vi "9024_8_9230.vi"() -> (2 "Device":T3={"Id"="55379f6619257936b04df56a", "Name"="Tms9024", "DeviceType"="CMS-9024", "HardwareName"="", "IpAddress"="10.2.64.47", "HardwareInfo"=[{"Key"="Controller", "Value"="cRIO 9024"}, {"Key"="Slot 1", "Value"="NI 9232 Tachometer"}, {"Key"="Slot 2", "Value"="NI 9230"}, {"Key"="Slot 3", "Value"="NI 9230"}, {"Key"="Slot 4", "Value"="NI 9230"}, {"Key"="Slot 5", "Value"="NI 9230"}, {"Key"="Slot 6", "Value"="NI 9230"}, {"Key"="Slot 7", "Value"="NI 9230"}, {"Key"="Slot 8", "Value"="NI 9230"}], "ApplicationType"="", "ApplicationVersion"="", "EquipmentIds"=[], "ConfigurationVersion"="2015-04-22T08:26:15.5019992-05:00", "ConfigurationBag"="", "Properties"=[{"Key"="FileMemoryTransferMode", "Value"="true"}, {"Key"="StreamMode", "Value"="InMemOrDisk"}, {"Key"="TdmsMemoryBlockSize", "Value"="8388608"}, {"Key"="TdmsMemoryStreamBlockSize", "Value"="1048576"}, {"Key"="ReconnectInterval", "Value"="30"}, {"Key"="PacketSizeKbytes", "Value"="16"}, {"Key"="InterPacketDelay", "Value"="0"}, {"Key"="FeatureSpeedCutoff", "Value"="120"}, {"Key"="SpeedReference", "Value"=""}, {"Key"="DataBlockLength", "Value"="4"}, {"Key"="DataBlockUnit", "Value"="Seconds"}, {"Key"="AcquisitionLength", "Value"="7"}, {"Key"="PreTriggerLength", "Value"="3"}, {"Key"="AcquisitionUnit", "Value"="Seconds"}], "DataGroups"=[{"Name"="Default", "ChannelIds"=["55379f6619257936b04df56b", "55379f6619257936b04df56e", "55379f6619257936b04df571", "55379f6619257936b04df574", "55379f6619257936b04df579", "55379f6619257936b04df57e"], "GatingTrigger"={"Type"="", "Expression"="", "Conditions"=[]}, "OperatingStates"=[{"Id"="55379f6619257936b04df59b", "Name"="SteadyState", "StreamMode"=FALSE, "EnterTrigger"={"Type"="", "Expression"="", "Conditions"=[]}, "ExitTrigger"={"Type"="", "Expression"="", "Conditions"=[]}, "TagCollectionTrigger"={"Type"="", "Expression"="", "Conditions"=[]}, "FileCollectionTrigger"={"Type"="", "Expression"="C1", "Conditions"=[{"Source"="Cron", "Type"="Cron", "Operator"="Greater", "CompareTo"="0 0,1,2,3,4,5,6,7,8,9,10,11,12,13,14,15,16,17,18,19,20,21,22,23 * * * *", "DwellSeconds"=0.0}]}, "Properties"=[{"Key"="AcquisitionLength", "Value"="7"}, {"Key"="PreTriggerLength", "Value"="3"}, {"Key"="AcquisitionUnit", "Value"="Seconds"}]}, {"Id"="55379f6619257936b04df59c", "Name"="Run-Up", "StreamMode"=TRUE, "EnterTrigger"={"Type"="", "Expression"="", "Conditions"=[{"Source"="55379f6619257936b04df583", "Type"="Double", "Operator"="GreaterIncreasing", "CompareTo"="200", "DwellSeconds"=0.0}]}, "ExitTrigger"={"Type"="", "Expression"="C1 OR C2 OR C3", "Conditions"=[{"Source"="55379f6619257936b04df583", "Type"="Double", "Operator"="Greater", "CompareTo"="1200", "DwellSeconds"=20.0}, {"Source"="55379f6619257936b04df59d", "Type"="TimespanSeconds", "Operator"="GreaterEqual", "CompareTo"="3600", "DwellSeconds"=0.0}, {"Source"="55379f6619257936b04df583", "Type"="Double", "Operator"="Less", "CompareTo"="200", "DwellSeconds"=20.0}]}, "TagCollectionTrigger"={"Type"="", "Expression"="", "Conditions"=[]}, "FileCollectionTrigger"={"Type"="", "Expression"="C1 OR C2", "Conditions"=[{"Source"="55379f6619257936b04df583", "Type"="Double", "Operator"="Delta", "CompareTo"="50", "DwellSeconds"=0.0}, {"Source"="55379f6619257936b04df59e", "Type"="TimespanSeconds", "Operator"="GreaterEqual", "CompareTo"="30", "DwellSeconds"=0.0}]}, "Properties"=[{"Key"="AcquisitionLength", "Value"="10"}, {"Key"="PreTriggerLength", "Value"="0"}, {"Key"="AcquisitionUnit", "Value"="Seconds"}]}, {"Id"="55379f6619257936b04df59f", "Name"="Coast-Down", "StreamMode"=TRUE, "EnterTrigger"={"Type"="", "Expression"="", "Conditions"=[{"Source"="55379f6619257936b04df583", "Type"="Double", "Operator"="LessDecreasing", "CompareTo"="1200", "DwellSeconds"=0.0}]}, "ExitTrigger"={"Type"="", "Expression"="C1 OR C2 OR C3", "Conditions"=[{"Source"="55379f6619257936b04df583", "Type"="Double", "Operator"="Less", "CompareTo"="200", "DwellSeconds"=20.0}, {"Source"="55379f6619257936b04df5a0", "Type"="TimespanSeconds", "Operator"="GreaterEqual", "CompareTo"="3600", "DwellSeconds"=0.0}, {"Source"="55379f6619257936b04df583", "Type"="Double", "Operator"="Greater", "CompareTo"="1200", "DwellSeconds"=20.0}]}, "TagCollectionTrigger"={"Type"="", "Expression"="", "Conditions"=[]}, "FileCollectionTrigger"={"Type"="", "Expression"="C1 OR C2", "Conditions"=[{"Source"="55379f6619257936b04df583", "Type"="Double", "Operator"="Delta", "CompareTo"="50", "DwellSeconds"=0.0}, {"Source"="55379f6619257936b04df5a1", "Type"="TimespanSeconds", "Operator"="GreaterEqual", "CompareTo"="30", "DwellSeconds"=0.0}]}, "Properties"=[{"Key"="AcquisitionLength", "Value"="10"}, {"Key"="PreTriggerLength", "Value"="0"}, {"Key"="AcquisitionUnit", "Value"="Seconds"}]}], "Properties"=[{"Key"="SpeedReference", "Value"="55379f6619257936b04df56b"}, {"Key"="DataBlockLength", "Value"="4"}, {"Key"="DataBlockUnit", "Value"="Seconds"}], "EquipmentIds"=[]}]}, 3 "system info":T1={"controller"={"vendorName"="National Instruments", "productName"="cRIO 9024", "serialNumber"="0183A6C6"}, "chassis"={"vendorName"="National Instruments", "productName"="NI cRIO-9114", "serialNumber"="01855B2D"}, "modules"=[{"vendorName"="National Instruments", "productName"="NI 9232", "serialNumber"="0182E2AC"}, {"vendorName"="National Instruments", "productName"="NI 9230", "serialNumber"="0185439C"}, {"vendorName"="", "productName"="NI 9230", "serialNumber"=""}, {"vendorName"="", "productName"="NI 9230", "serialNumber"=""}, {"vendorName"="", "productName"="NI 9230", "serialNumber"=""}, {"vendorName"="", "productName"="NI 9230", "serialNumber"=""}, {"vendorName"="", "productName"="NI 9230", "serialNumber"=""}, {"vendorName"="", "productName"="NI 9230", "serialNumber"=""}]})   [LabVIEW 2017]
uses:
  <vilib>/addons/InsightCM/MessageBus/Base/controls/KeyValuePair.ctl
  <vilib>/addons/InsightCM/MessageBus/Base/KeyValuePairs.ctl
  <vilib>/addons/InsightCM/MessageBus/Base/controls/Condition.ctl
  <vilib>/addons/InsightCM/MessageBus/Base/controls/Trigger.ctl
  <vilib>/addons/InsightCM/MessageBus/Base/controls/OperatingState.ctl
  <vilib>/addons/InsightCM/MessageBus/Base/controls/DataGroup.ctl
  <vilib>/addons/InsightCM/MessageBus/Base/controls/Device.ctl
  <vilib>/addons/cRIODetectHW/control/cRIO Product Info.ctl
  <vilib>/addons/cRIODetectHW/cRIODetectHW.lvlib
  <vilib>/addons/cRIODetectHW/control/SystemHW.ctl
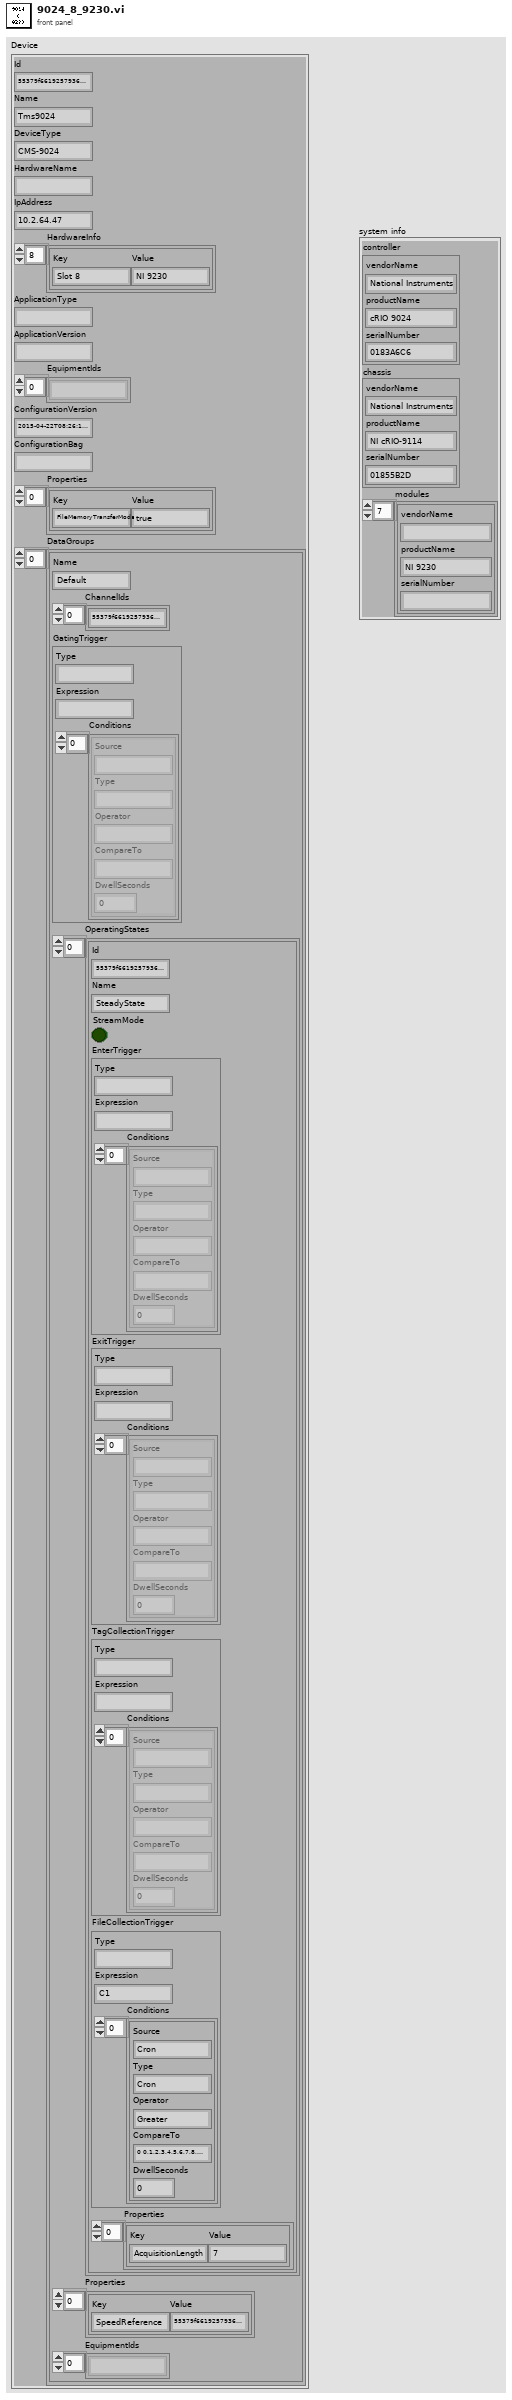
[diagram p1: front panel]
types:
  T1 = typedef "cRIODetectHW.lvlib/SystemHW.ctl" = cluster{"controller":T2, "chassis":T2, "modules":T2[]}
  T2 = typedef "cRIODetectHW.lvlib/cRIO Product Info.ctl" = cluster{"vendorName":string, "productName":string, "serialNumber":string}
  T3 = typedef "Device.ctl" = cluster{"Id":string, "Name":string, "DeviceType":string, "HardwareName":string, "IpAddress":string, "HardwareInfo":T4, "ApplicationType":string, "ApplicationVersion":string, "EquipmentIds":string[], "ConfigurationVersion":string, "ConfigurationBag":string, "Properties":T4, "DataGroups":T6[]}
  T4 = typedef "KeyValuePairs.ctl" = T5[]
  T5 = typedef "KeyValuePair.ctl" = cluster{"Key":string, "Value":string}
  T6 = typedef "DataGroup.ctl" = cluster{"Name":string, "ChannelIds":string[], "GatingTrigger":T7, "OperatingStates":T9[], "Properties":T4, "EquipmentIds":string[]}
  T7 = typedef "Trigger.ctl" = cluster{"Type":string, "Expression":string, "Conditions":T8[]}
  T8 = typedef "Condition.ctl" = cluster{"Source":string, "Type":string, "Operator":string, "CompareTo":string, "DwellSeconds":dbl}
  T9 = typedef "OperatingState.ctl" = cluster{"Id":string, "Name":string, "StreamMode":bool, "EnterTrigger":T7, "ExitTrigger":T7, "TagCollectionTrigger":T7, "FileCollectionTrigger":T7, "Properties":T4}
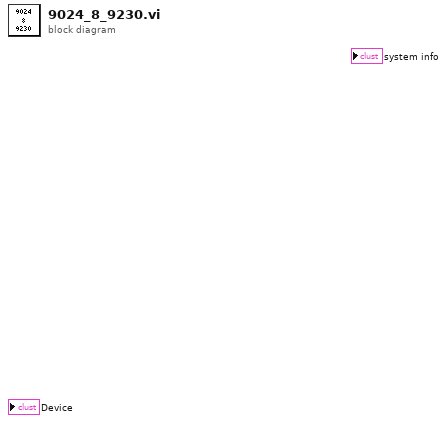
[diagram p0: block diagram]
diagram:
